vi "chart series set name range lv.vi"(7 "col":u16, 8 "error in (no error)":errorcluster, 9 "row":u32, 10 "sheetname":string, 11 "series":u32) -> (0 "error out":errorcluster)   [LabVIEW 8.6]
doc: "void chart_series_set_name_range_lv(lxw_chart_series series, const char *sheetname, lxw_row_t row, lxw_col_t col);"
uses:
  pending_lvxlsxwriter/xlsxwriter.dll
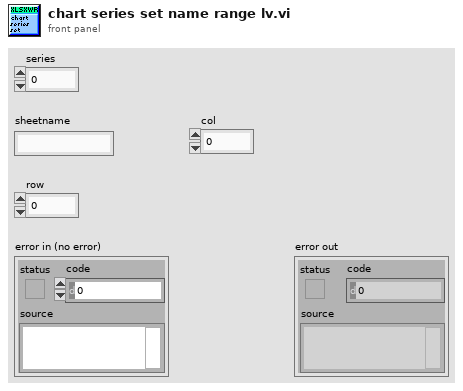
[diagram p1: front panel]
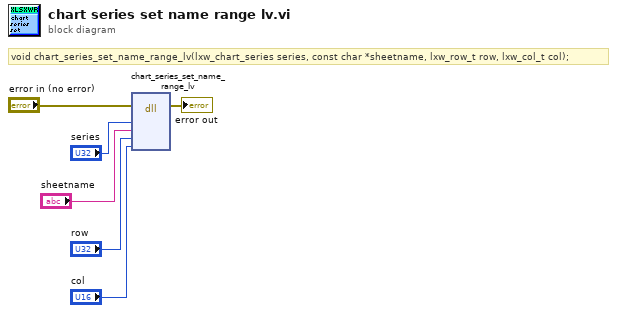
[diagram p0: block diagram]
diagram:
  # "void chart_series_set_name_range_lv(lxw_chart_series series, const char *sheetname, lxw_row_t row, lxw_col_t col);"
  n1 = dll-call lib="C:/Users/WDAGUtilityAccount/Desktop/pending_lvxlsxwriter/xlsxwriter.*" fn="chart_series_set_name_range_lv"(error in="error in (no error)", "series"="series", "sheetname"="sheetname", "row"="row", "col"="col") -> (error out=→"error out":errorcluster)  [unwired: 7 in, 1 out]
